vi "LS330_Set_SetP.vi"(7 "error in":errorcluster, 8 "Set Temp (K)":dbl, 9 "Heater":string(combo)="1", 10 "VISA resource name":refnum<visa-resource-name>) -> (0 "error out":errorcluster, 3 "VISA resource name out":refnum<visa-resource-name>)   [LabVIEW 2021]
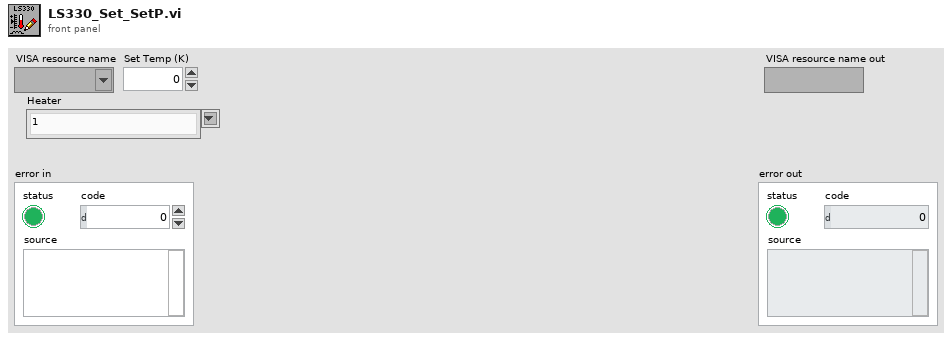
[diagram p1: front panel]
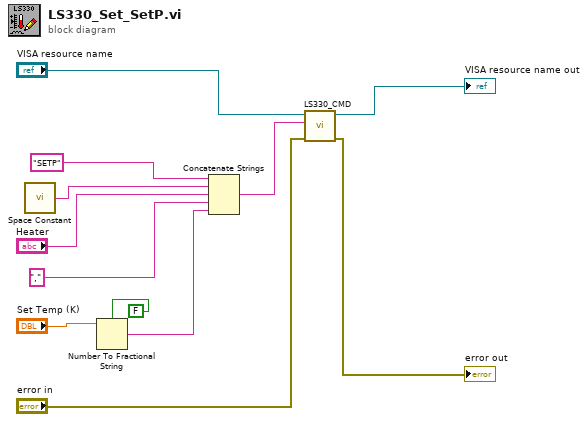
[diagram p0: block diagram]
diagram:
  n1 = call <vilib>:"Space Constant.vi"() -> ("String"=w10:string)
  n2 = Number To Fractional String(use system decimal point (T)=FALSE, number="Set Temp (K)") -> (F-format string=w3:string)  [unwired: 2 in]
  n3 = Concatenate Strings("SETP" ("string"), w10, "Heater", ",", w3) -> (w8:string)
  n4 = call "LS330_CMD.vi"("error in"="error in", "CMD"=w8, "VISA resource name"="VISA resource name") -> ("error out"=→"error out":errorcluster, "VISA resource name out"=→"VISA resource name out":refnum<visa-resource-name>)  [unwired: 7 in]
